vi "Launcher.vi"   [LabVIEW 2018]
uses:
  Server/Server/Server.lvclass
  C:/Program Files (x86)/National Instruments/LabVIEW 2018/vi.lib/ActorFramework/Actor/Actor.lvclass
  <vilib>/ActorFramework/Actor/Actor.lvclass
panel:
  # "Actor Chat Window - Launcher!\nTom's LabVIEW Adventure\nhttps://www.youtube.com/tomslabviewadventure"
types:
  T1 = enum32{"Invalid", "Standard", "Closed", "Hidden", "Minimized", "Maximized"}
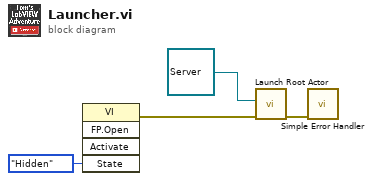
[diagram p0: block diagram]
diagram:
  n1 = invoke class="VI" method="FP.Open"("State"=T1."Hidden") -> (error out=w2:errorcluster)  [unwired: 4 in, 4 out]
  n2 = call <vilib>:"Launch Root Actor.vi"("error in (no error)"=w2, "Actor"=refnum<class "Server.lvclass"> refnum ("Server.lvlib:Server.lvclass")) -> ("error out"=w1:errorcluster)  [unwired: 8 in, 1 out]
  n3 = call <vilib>:"Simple Error Handler.vi"("error in (no error)"=w1) -> ()  [unwired: 4 in, 5 out]
